vi "String Label.vi"(9 "i":i64, 10 "Input String":string) -> (2 "resulting string":string)   [LabVIEW 2019, in "Transport.lvclass"]
uses:
  Transport.lvclass
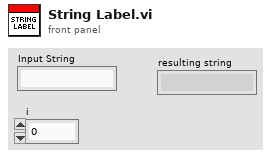
[diagram p1: front panel]
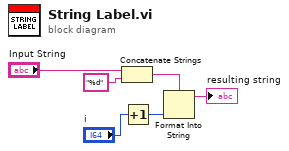
[diagram p0: block diagram]
diagram:
  n1 = Concatenate Strings("Input String", "%d" ("wavenames")) -> (w4:string)
  n2 = Increment(x="i") -> (x+1=w3:i64)
  n3 = Format Into String(format string=w4, w3) -> (resulting string=→"resulting string":string)  [unwired: 2 in, 1 out]
